vi "Replace Control.vi"(0 "VI in":refnum<vi>, 5 "JSON String":string, 7 "Control in":refnum<vi>, 11 "error in (no error)":errorcluster) -> (4 "VI out":refnum<vi>, 8 "Control out":refnum<vi>, 15 "error out":errorcluster)   [LabVIEW 2017]
uses:
  Advanced LabVIEW Variant APIs/Advanced Variant Tools.lvlib
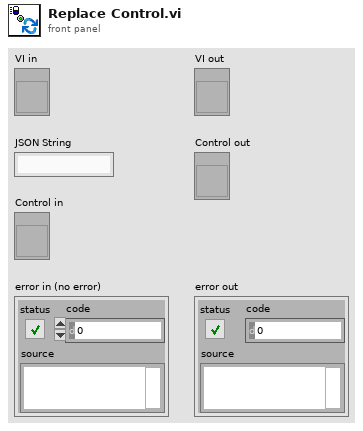
[diagram p1: front panel]
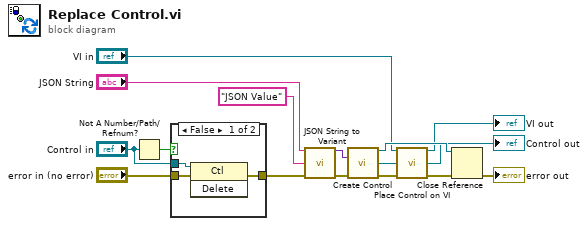
[diagram p0: block diagram]
diagram:
  n1 = Not A Number/Path/Refnum?(number/path/refnum="Control in") -> (NaN/Path/Refnum?=w4:bool)
  n2 = case shown="False" w4 {
    tunnel: "Control in" -> [w19 _]
    tunnel: "error in (no error)" -> [w18 w20]
    tunnel: [w17 w20] -> w1
    frame False {
      n3 = invoke class="Ctl" method="Delete"(reference=w19, error in=w18) -> (error out=w17:errorcluster)  [unwired: 1 in, 2 out]
    }
    frame True {
    }
  }
  n4 = call "JSON String to Variant.vi"("JSON String"="JSON String", "Top-Level Control Name"="JSON Value", "error in (no error)"=w1) -> ("Variant out"=w7:variant, "error out"=w8:errorcluster)  [unwired: 11 in]
  n5 = call "Create Control.vi"("Variant in"=w7, "error in (no error)"=w8) -> ("Control VI out"=w16:refnum<vi>, "Control Reference out"=w13:refnum<vi>, "error out"=w9:errorcluster)  [unwired: 11 in]
  n6 = call "Place Control on VI.vi"("VI in"="VI in", "Control in"=w13, "error in (no error)"=w9) -> ("VI out"=→"VI out":refnum<vi>, "Control out"=→"Control out":refnum<vi>, "error out"=w10:errorcluster)  [unwired: 10 in]
  n7 = Close Reference(reference=w16, error in (no error)=w10) -> (error out=→"error out":errorcluster)
